vi "Main.vi"() -> ()   [LabVIEW 2013]
doc: "本模板用于队列消息处理器设计模式。\n\n事件处理循环负责按用户界面操作生成对应的消息。\n\n消息处理循环负责对事件处理循环或其他消息生成的消息进行处理。消息内容为字符串值，因此很容易将新消息添加至“消息处理”循环的“消息分支”条件结构。每个消息簇还可选择性地为消息数据提供一个变体，变体数据可以转换为消息数据所需要的任意类型。"
uses:
  controls/UI Data.ctl
  support/Message Queue/Enqueue Message (Single).vi
  support/Message Queue/Enqueue Message (Array).vi
  <vilib>/Utility/error.llb/Error Cluster From Error Code.vi
  <vilib>/ErrorRing/Error Ring.xnode
  support/Message Queue/Message Queue.lvlib
  support/User Event - Stop/User Event - Stop.lvlib
panel:
  out "显示<替换该项>":string
  in  "执行其他操作<替换该项>":bool
  in  "执行某操作<替换该项>":bool
  in  "退出":bool
  # "这些控件和“值改变”事件关联，通过程序框图中的事件结构配置。\n\n按应用程序的实际需求，将这些控件替换为所需控件，并对事件结构重新配置。"
  # "本模板用于队列消息处理器设计模式。\n\n关于本模板用法的更多信息，见程序框图。"
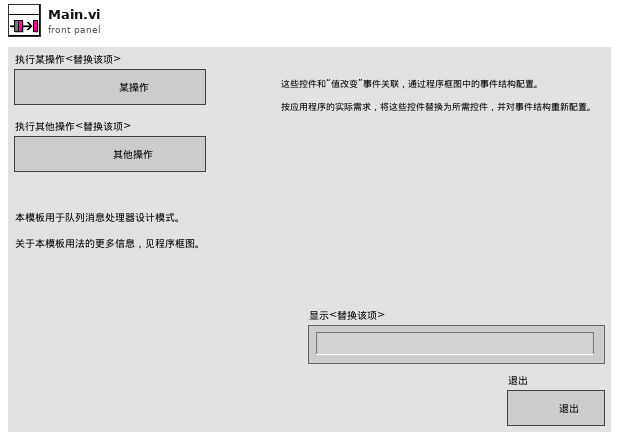
[diagram p1: front panel]
types:
  T1 = typedef "UI Data.ctl" = cluster{"布尔<替换该项>":bool, "字符串<替换该项>":string, "数值<替换该项>":dbl, "执行某操作引用":refnum<vi>, "执行其他操作引用":refnum<vi>, "数据显示引用":refnum<vi>, "退出按钮引用":refnum<vi>}
  T2 = typedef "Message Queue.lvlib/All Message Queues.ctl" = cluster{"UI":refnum<queue>}
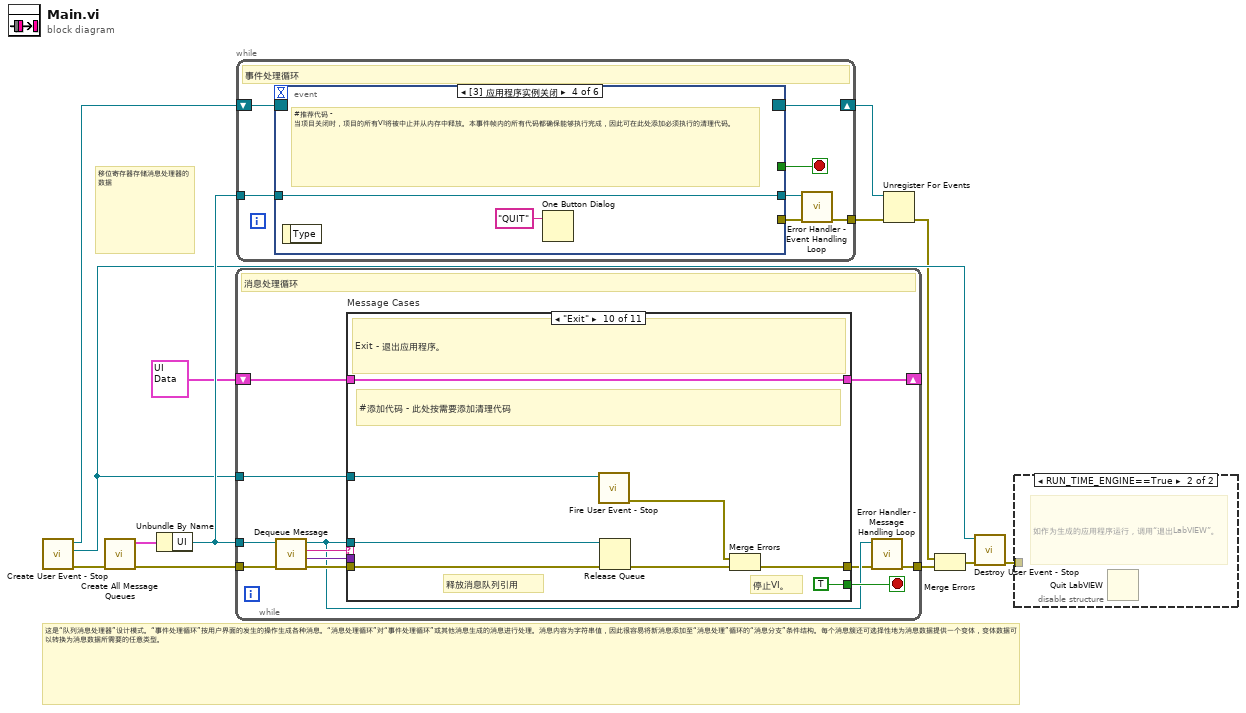
[diagram p0: block diagram]
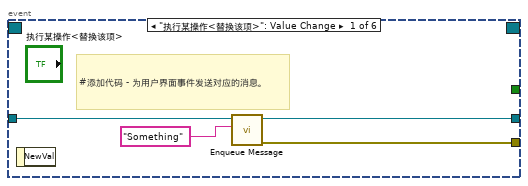
[diagram p3: hidden frame]
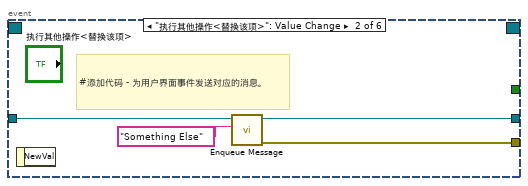
[diagram p4: hidden frame]
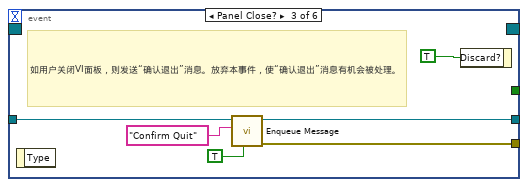
[diagram p5: hidden frame]
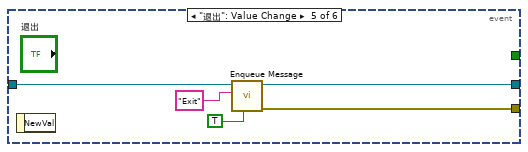
[diagram p6: hidden frame]
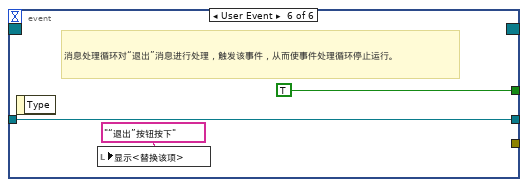
[diagram p7: hidden frame]
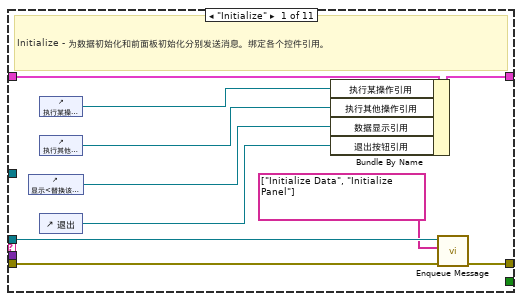
[diagram p8: hidden frame]
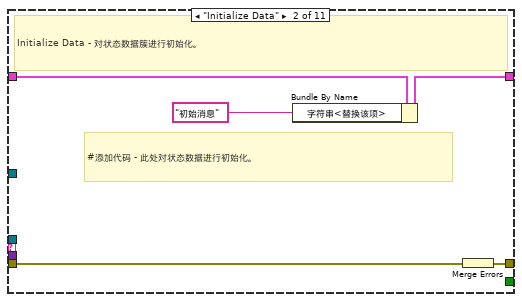
[diagram p9: hidden frame]
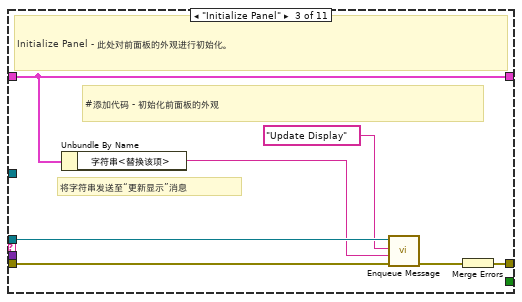
[diagram p10: hidden frame]
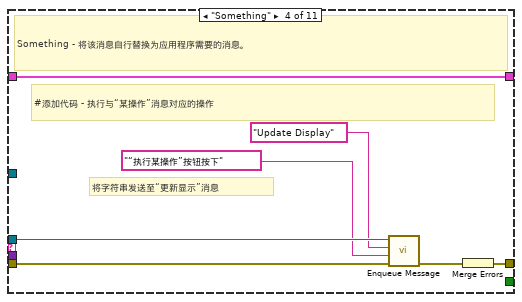
[diagram p11: hidden frame]
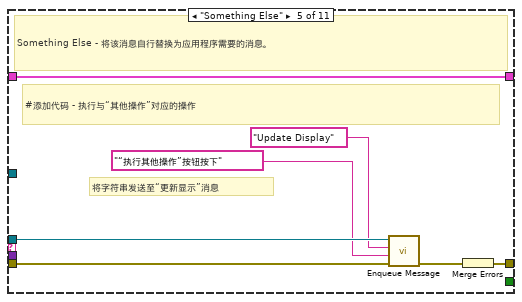
[diagram p12: hidden frame]
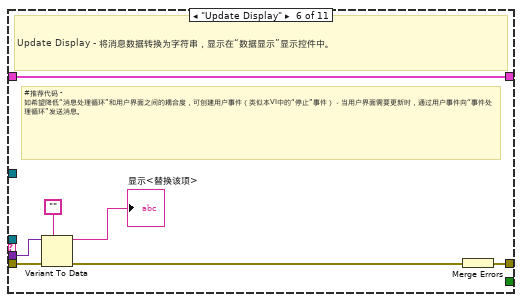
[diagram p13: hidden frame]
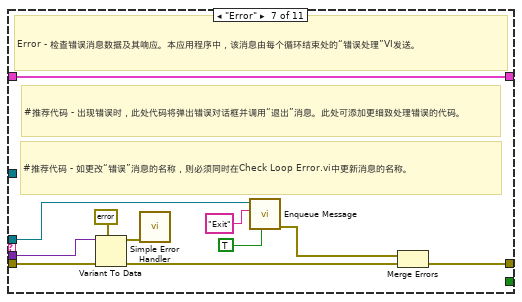
[diagram p14: hidden frame]
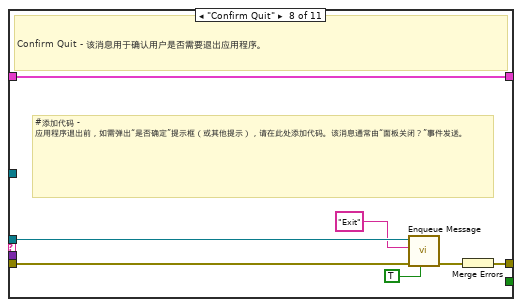
[diagram p15: hidden frame]
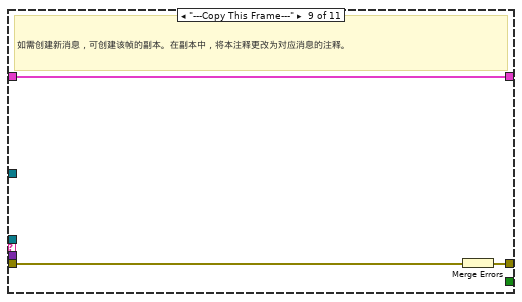
[diagram p16: hidden frame]
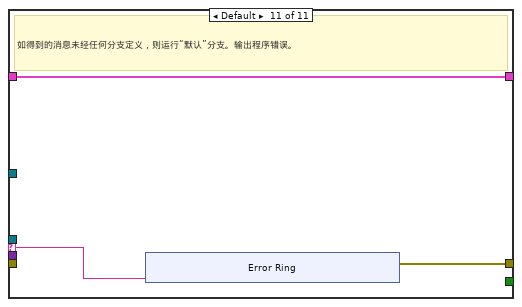
[diagram p17: hidden frame]
diagram:
  # "这是“队列消息处理器”设计模式。“事件处理循环”按用户界面的发生的操作生成各种消息。“消息处理循环”对“事件处理循环”或其他消息生成的消息进行处理。消息内容为字符串值，因此很容易将新消息添加至“消息处理”循环的“消息分支”条件结构。每个消息簇还可选择性地为消息数据提供一个变体，变体数据可以转换为消息数据所需要的任意类型。"
  # "移位寄存器存储消息处理器的数据"
  n1 = call "Create User Event - Stop.vi"() -> ("error out"=w8:cluster{"状态":bool, "代码":i32, "源":string}, "用户事件－停止"=w6:refnum<user-event>, "停止事件注册引用句柄"=w9:refnum<event-registration>)  [unwired: 9 in]
  n2 = call "Create All Message Queues.vi"("error in (no error)"=w8) -> ("error out"=w13:cluster{"状态":bool, "代码":i32, "源":string}, "消息队列输出"=w12:T2)  [unwired: 9 in]
  n3 = Unbundle By Name(w12) -> ("UI"=w10:refnum<queue>)
  n4 = while {
    tunnel: w10 -> [w17]
    shift-right: [w24] -> _
    shift-left: T1 {"布尔<替换该项>"=FALSE, "字符串<替换该项>"="", "数值<替换该项>"=0.0, "执行某操作引用"=refnum, "执行其他操作引用"=refnum, "数据显示引用"=refnum, "退出按钮引用"=refnum} ("Data Cluster") -> [w25]
    tunnel: w6 -> [w22]
    tunnel: w13 -> [w21]
    tunnel: [w15] -> w11
    stop <- w23 stop-if-true
    # "消息处理循环"
    n5 = call "Dequeue Message.vi"("error in (no error)"=w21, "消息队列"=w17) -> ("error out"=w20:cluster{"状态":bool, "代码":i32, "源":string}, "消息数据"=w18:variant, "消息"=w19:string, "消息队列副本"=w16:refnum<queue>)  [unwired: 6 in]
    n6 = case "Message Cases" shown="\"Exit\"" w19 {
      selector: w19 -> [_ _ _ _ _ _ _ _ _ _ w98]
      tunnel: w16 -> [w33 _ w44 w50 w57 _ w71 w82 _ w97 _]
      tunnel: w20 -> [w34 w40 w45 w52 w59 w66 w79 w86 w89 w92 _]
      tunnel: [w35 w36 w46 w53 w60 w67 w72 w84 w87 w93 w99] -> w14
      tunnel: w25 -> [w32 w39 w47 w54 w61 w68 w78 w85 w88 w96 w100]
      tunnel: [w31 w38 w47 w54 w61 w68 w78 w85 w88 w96 w100] -> w24
      tunnel: [_ _ _ _ _ _ _ _ _ TRUE _] -> w23
      tunnel: w18 -> [_ _ _ _ _ w65 w77 _ _ _ _]
      tunnel: w22 -> [_ _ _ _ _ _ _ _ _ w91 _]
      frame "Initialize" {
        # "Initialize - 为数据初始化和前面板初始化分别发送消息。绑定各个控件引用。"
        n7 = control-ref of="显示<替换该项>"() -> (w28:refnum<vi>)
        n8 = control-ref of="执行某操作<替换该项>"() -> (w30:refnum<vi>)
        n9 = control-ref of="执行其他操作<替换该项>"() -> (w29:refnum<vi>)
        n10 = control-ref of="退出"() -> (w27:refnum<vi>)
        n11 = Bundle By Name(cluster=w32, "执行某操作引用"=w30, "执行其他操作引用"=w29, "数据显示引用"=w28, "退出按钮引用"=w27) -> (w31:T1)
        n12 = call-poly "Enqueue Message.vi"("error in (no error)"=w34, "消息数组"=string[] ["Initialize Data", "Initialize Panel"], "消息队列"=w33) -> ("error out"=w35:cluster{"状态":bool, "代码":i32, "源":string})  [unwired: 7 in, 1 out]
      }
      frame "Initialize Data" {
        # "#添加代码 - 此处对状态数据进行初始化。"
        # "Initialize Data - 对状态数据簇进行初始化。"
        n13 = Bundle By Name(cluster=w39, "字符串<替换该项>"="初始消息" ("Initial Message")) -> (w38:T1)
        n14 = Merge Errors(w40) -> (w36:errorcluster)
      }
      frame "Initialize Panel" {
        # "将字符串发送至“更新显示”消息"
        # "#添加代码 - 初始化前面板的外观"
        # "Initialize Panel - 此处对前面板的外观进行初始化。"
        n15 = Unbundle By Name(w47) -> ("字符串<替换该项>"=w41:string)
        n16 = call-poly "Enqueue Message.vi"("error in (no error)"=w45, "消息数据"=w41, "消息"="Update Display" ("Message"), "消息队列"=w44) -> ("error out"=w43:cluster{"状态":bool, "代码":i32, "源":string})  [unwired: 6 in, 1 out]
        n17 = Merge Errors(w43) -> (w46:errorcluster)
      }
      frame "Something" {
        # "将字符串发送至“更新显示”消息"
        # "#添加代码 - 执行与“某操作”消息对应的操作"
        # "Something - 将该消息自行替换为应用程序需要的消息。"
        n18 = call-poly "Enqueue Message.vi"("error in (no error)"=w52, "消息数据"="“执行某操作”按钮按下" ("\"Do Something\" button pressed"), "消息"="Update Display" ("Message"), "消息队列"=w50) -> ("error out"=w51:cluster{"状态":bool, "代码":i32, "源":string})  [unwired: 6 in, 1 out]
        n19 = Merge Errors(w51) -> (w53:errorcluster)
      }
      frame "Something Else" {
        # "将字符串发送至“更新显示”消息"
        # "#添加代码 - 执行与“其他操作”对应的操作"
        # "Something Else - 将该消息自行替换为应用程序需要的消息。"
        n20 = call-poly "Enqueue Message.vi"("error in (no error)"=w59, "消息数据"="“执行其他操作”按钮按下" ("\"Do Something Else\" button pressed"), "消息"="Update Display" ("Message"), "消息队列"=w57) -> ("error out"=w58:cluster{"状态":bool, "代码":i32, "源":string})  [unwired: 6 in, 1 out]
        n21 = Merge Errors(w58) -> (w60:errorcluster)
      }
      frame "Update Display" {
        # "#推荐代码 - 如希望降低“消息处理循环”和用户界面之间的耦合度，可创建用户事件（类似本VI中的“停止”事件）－当用户界面需要更新时，通过用户事件向“事件处理循环”发送消息。"
        # "Update Display - 将消息数据转换为字符串，显示在“数据显示”显示控件中。"
        n22 = Variant To Data(error in=w66, type="", Variant=w65) -> (data=→"显示<替换该项>":string, error out=w63:errorcluster)
        n23 = Merge Errors(w63) -> (w67:errorcluster)
      }
      frame "Error" {
        # "#推荐代码 - 如更改“错误”消息的名称，则必须同时在Check Loop Error.vi中更新消息的名称。"
        # "#推荐代码 - 出现错误时，此处代码将弹出错误对话框并调用“退出”消息。此处可添加更细致处理错误的代码。"
        # "Error - 检查错误消息数据及其响应。本应用程序中，该消息由每个循环结束处的“错误处理”VI发送。"
        n24 = Variant To Data(error in=w79, type=errorcluster {"status"=FALSE, "code"=0, "source"=""} ("error constant"), Variant=w77) -> (data=w75:errorcluster, error out=w74:errorcluster)
        n25 = call <vilib>:"Simple Error Handler.vi"("error in (no error)"=w75) -> ()  [unwired: 4 in, 5 out]
        n26 = call-poly "Enqueue Message.vi"("优先消息？(F)"=TRUE ("Priority Message? (F)"), "消息"="Exit", "消息队列"=w71) -> ("error out"=w73:cluster{"状态":bool, "代码":i32, "源":string})  [unwired: 7 in, 1 out]
        n27 = Merge Errors(w73, w74) -> (w72:errorcluster)
      }
      frame "Confirm Quit" {
        # "#添加代码 - 应用程序退出前，如需弹出“是否确定”提示框（或其他提示），请在此处添加代码。该消息通常由“面板关闭？”事件发送。"
        # "Confirm Quit - 该消息用于确认用户是否需要退出应用程序。"
        n28 = call-poly "Enqueue Message.vi"("优先消息？(F)"=TRUE ("Priority Message? (F)"), "error in (no error)"=w86, "消息"="Exit" ("Message"), "消息队列"=w82) -> ("error out"=w83:cluster{"状态":bool, "代码":i32, "源":string})  [unwired: 6 in, 1 out]
        n29 = Merge Errors(w83) -> (w84:errorcluster)
      }
      frame "---Copy This Frame---" {
        # "如需创建新消息，可创建该帧的副本。在副本中，将本注释更改为对应消息的注释。"
        n30 = Merge Errors(w89) -> (w87:errorcluster)
      }
      frame "Exit" {
        # "停止VI。"
        # "释放消息队列引用"
        # "#添加代码 - 此处按需要添加清理代码"
        # "Exit - 退出应用程序。"
        n31 = call "Fire User Event - Stop.vi"("用户事件－停止"=w91) -> ("error out"=w90:cluster{"状态":bool, "代码":i32, "源":string})  [unwired: 10 in]
        n32 = Release Queue(queue=w97, error in (no error)=w92) -> (error out=w94:errorcluster)  [unwired: 1 in, 2 out]
        n33 = Merge Errors(w90, w94) -> (w93:errorcluster)
      }
      frame Default {
        # "如得到的消息未经任何分支定义，则运行“默认”分支。输出程序错误。"
        n34 = xnode "Error Ring"("参数 0"=w98) -> ("错误输出"=w99:errorcluster)
      }
    }
    n35 = call "Error Handler - Message Handling Loop.vi"("error in (no error)"=w14, "消息队列"=w16) -> ("错误输入副本"=w15:cluster{"状态":bool, "代码":i32, "源":string})  [unwired: 8 in, 1 out]
  }
  n36 = while {
    tunnel: w10 -> [w114]
    shift-right: [w112] -> w4
    shift-left: w9 -> [w113]
    tunnel: [w108] -> w1
    stop <- w110 stop-if-true
    # "事件处理循环"
    n37 = event shown="[3] 应用程序实例关闭" {
      selector: w113 -> [_ _ _ _ _ _]
      dyn-events: [_ _ _ _ _ _] -> w112
      timeout: _ -> [_ _ _ _ _ _]
      tunnel: [_ _ _ _ _ TRUE ("Discard?")] -> w110
      tunnel: w114 -> [w118 w122 w127 w130 w135 w138]
      tunnel: [w115 w119 w126 _ w134 _] -> w111
      tunnel: [w117 w121 w125 w130 w133 w138] -> w109
      event "执行某操作<替换该项>": Value Change {
        # "#添加代码 - 为用户界面事件发送对应的消息。"
        n38 = event-data() -> ()  [unwired: 1 in, 1 out]
        n39 = call-poly "Enqueue Message.vi"("消息"="Something" ("Message"), "消息队列"=w118) -> ("error out"=w115:cluster{"状态":bool, "代码":i32, "源":string}, "消息队列副本"=w117:refnum<queue>)  [unwired: 8 in]
      }
      event "执行其他操作<替换该项>": Value Change {
        # "#添加代码 - 为用户界面事件发送对应的消息。"
        n40 = event-data() -> ()  [unwired: 1 in, 1 out]
        n41 = call-poly "Enqueue Message.vi"("消息"="Something Else" ("Message"), "消息队列"=w122) -> ("error out"=w119:cluster{"状态":bool, "代码":i32, "源":string}, "消息队列副本"=w121:refnum<queue>)  [unwired: 8 in]
      }
      event Panel Close? {
        # "如用户关闭VI面板，则发送“确认退出”消息。放弃本事件，使“确认退出”消息有机会被处理。"
        n42 = event-data() -> ()  [unwired: 1 in, 1 out]
        n43 = call-poly "Enqueue Message.vi"("优先消息？(F)"=TRUE ("Priority Message? (F)"), "消息"="Confirm Quit" ("Message"), "消息队列"=w127) -> ("error out"=w126:cluster{"状态":bool, "代码":i32, "源":string}, "消息队列副本"=w125:refnum<queue>)  [unwired: 7 in]
        n44 = event-data("Discard?"=TRUE) -> ()  [unwired: 1 in, 1 out]
      }
      event Application Instance Close {
        # "#推荐代码 - 当项目关闭时，项目的所有VI将被中止并从内存中释放。本事件帧内的所有代码都确保能够执行完成，因此可在此处添加必须执行的清理代码。"
        n45 = event-data() -> ()  [unwired: 1 in, 1 out]
        n46 = One Button Dialog(message="QUIT" ("消息")) -> ()  [unwired: 1 in, 1 out]
      }
      event "退出": Value Change {
        n47 = event-data() -> ()  [unwired: 1 in, 1 out]
        n48 = call-poly "Enqueue Message.vi"("优先消息？(F)"=TRUE ("Priority Message? (F)"), "消息"="Exit" ("Message"), "消息队列"=w135) -> ("error out"=w134:cluster{"状态":bool, "代码":i32, "源":string}, "消息队列副本"=w133:refnum<queue>)  [unwired: 7 in]
      }
      event User Event {
        # "消息处理循环对“退出”消息进行处理，触发该事件，从而使事件处理循环停止运行。"
        n49 = event-data() -> ()  [unwired: 1 in, 1 out]
        n50 = local write "显示<替换该项>"("“退出”按钮按下" ("VI Stopped")) -> ()
      }
    }
    n51 = call "Error Handler - Event Handling Loop.vi"("error in (no error)"=w111, "消息队列"=w109) -> ("错误输入副本"=w108:cluster{"状态":bool, "代码":i32, "源":string})  [unwired: 8 in, 1 out]
  }
  n52 = Unregister For Events(event registration refnum=w4, error in=w1) -> (error out=w5:errorcluster)
  n53 = Merge Errors(w5, w11) -> (w7:errorcluster)
  n54 = call "Destroy User Event - Stop.vi"("error in (no error)"=w7, "用户事件－停止"=w6) -> ("error out"=w2:cluster{"状态":bool, "代码":i32, "源":string})  [unwired: 9 in]
  n55 = disable-structure shown="RUN_TIME_ENGINE==True" {
    disable-tunnel: w2 -> [_ _]
    frame condition #0 (active) {
    }
    frame condition #1 {
      # "如作为生成的应用程序运行，调用“退出LabVIEW”。"
      n56 = Quit LabVIEW() -> ()  [unwired: 1 in]
    }
  }
